vi "Tag Frames.vi"(5 "Single Channel Select":T5(ring), 6 "Frame Tag Bypass":T1, 7 "Enable Frame Tagging":bool, 8 "Input Valid":bool, 9 "Line Status In":T3, 10 "DC Overvoltage":bool, 11 "Data In":i16[](array[numeric])=[0, 0, 0, 0]) -> (1 "Line Status Out":T3, 3 "Data":T4, 4 "Frames Acquired":u32)   [LabVIEW 2014]
uses:
  Acquisition Engine/Acquisition Status.ctl
  Async Frametag Data.ctl
panel:
  # "Copyright 2014 Vidrio Technologies\nScanImage 5 software is licensed under the Apache License, Version 2.0 (the \"License\"); you may not use any files contained\nwithin the ScanImage 5 release except in compliance with the License. You may obtain a copy of the License at\n http://www.apache.org/licenses/LICENSE-2.0\nUnless required by applicable law or agreed to in writing, software distributed under the License is distributed on an\n\"AS IS\" BASIS, WITHOUT WARRANTIES OR CONDITIONS OF ANY KIND, either express or implied. See the License for the\n specific language governing permissions and limitations under the License."
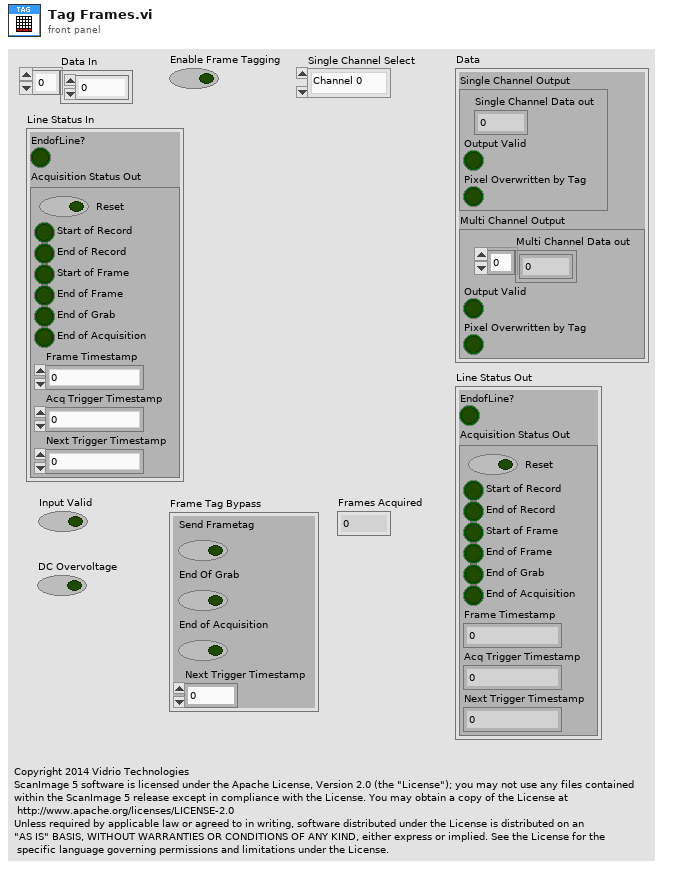
[diagram p1: front panel]
types:
  T1 = typedef "Async Frametag Data.ctl" = cluster{"Send Frametag":bool, "End Of Grab":bool, "End of Acquisition":bool, "Next Trigger Timestamp":u64}
  T2 = typedef "Acquisition Status.ctl" = cluster{"Reset":bool, "Start of Record":bool, "End of Record":bool, "Start of Frame":bool, "End of Frame":bool, "End of Grab":bool, "End of Acquisition":bool, "Frame Timestamp":u64, "Acq Trigger Timestamp":u64, "Next Trigger Timestamp":u64}
  T3 = cluster{"EndofLine?":bool, "Acquisition Status Out":T2}
  T4 = cluster{"Single Channel Output":cluster{"Single Channel Data out":i16, "Output Valid":bool, "Pixel Overwritten by Tag":bool}, "Multi Channel Output":cluster{"Multi Channel Data out":i16[], "Output Valid":bool, "Pixel Overwritten by Tag":bool}}
  T5 = enum8{"Channel 0", "Channel 1", "Channel 2", "Channel 3"}
  T6 = cluster{"Multi Channel Data out":i16[], "Output Valid":bool, "Pixel Overwritten by Tag":bool}
  T7 = cluster{"Single Channel Data out":i16, "Output Valid":bool, "Pixel Overwritten by Tag":bool}
  T8 = typedef "Frametag Data.ctl" = cluster{"Acquisition Status Flags":u16, "Frame Number":u32, "Frame Timestamp":u64, "Acq Trigger Timestamp":u64, "Next Trigger Timestamp":u64}
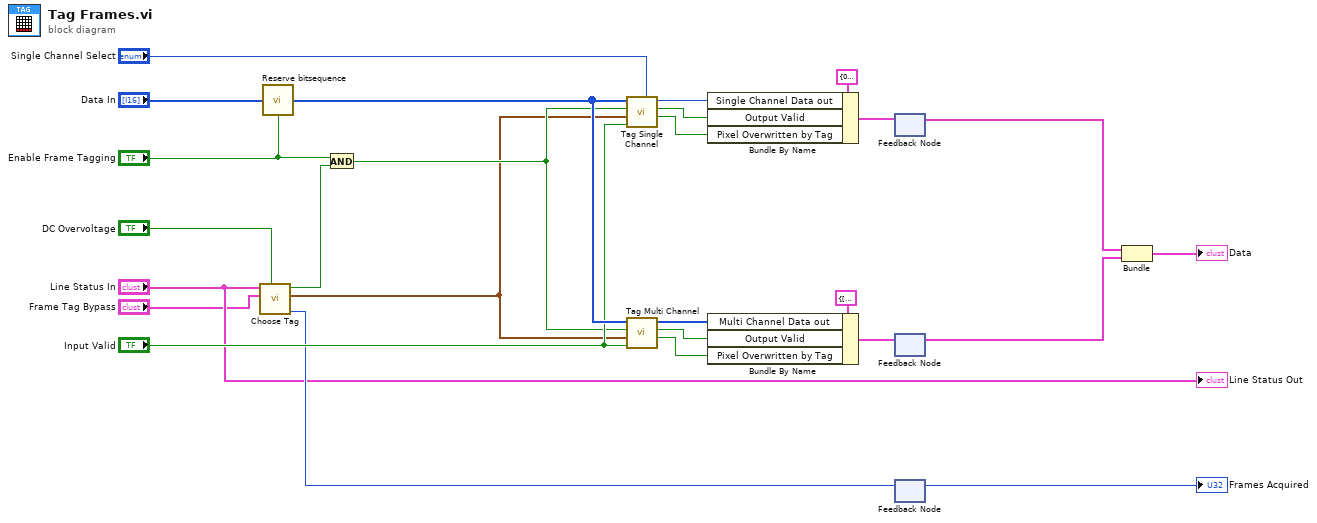
[diagram p0: block diagram]
diagram:
  n1 = call "Choose Tag.vi"("DC Overvoltage"="DC Overvoltage", "Frame Tag Bypass"="Frame Tag Bypass", "Line Status In"="Line Status In") -> ("Frame Count"=w8:u32, "Frametag Data"=w1:T8, "Send Tag"=w3:bool)  [unwired: 6 in]
  n2 = call "Reserve bitsequence.vi"("Data in"="Data In", "Reserve bitsequence"="Enable Frame Tagging") -> ("Data out"=w26:i16[])  [unwired: 13 in]
  n3 = And(x="Enable Frame Tagging", y=w3) -> (x .and. y?=w2:bool)
  n4 = call "Tag Single Channel.vi"("Data in"=w26, "Tag Record"=w2, "TagData"=w1, "Input Valid"="Input Valid", "Channel"="Single Channel Select") -> ("Single Channel Data out"=w22:i16, "Output Valid"=w21:bool, "Pixel Overwritten by Tag"=w23:bool)  [unwired: 3 in]
  n5 = call "Tag Multi Channel.vi"("Data in"=w26, "Tag Record"=w2, "TagData"=w1, "Input Valid"="Input Valid") -> ("Data out"=w18:i16[], "Output Valid"=w17:bool, "Pixel Overwritten"=w16:bool)  [unwired: 4 in]
  n6 = Bundle By Name(cluster=T7 {"Single Channel Data out"=0, "Output Valid"=FALSE, "Pixel Overwritten by Tag"=FALSE} ("Single Channel Output"), "Single Channel Data out"=w22, "Output Valid"=w21, "Pixel Overwritten by Tag"=w23) -> (w14:T7)
  n7 = Bundle By Name(cluster=T6 {"Multi Channel Data out"=[0, 0, 0, 0], "Output Valid"=FALSE, "Pixel Overwritten by Tag"=FALSE} ("Multi Channel Output"), "Multi Channel Data out"=w18, "Output Valid"=w17, "Pixel Overwritten by Tag"=w16) -> (w15:T6)
  n8 = feedback-in #1(w14) -> ()
  n9 = feedback #1() -> (w13:T7)  [unwired: 1 in]
  n10 = feedback #2() -> (w12:T6)  [unwired: 1 in]
  n11 = feedback-in #2(w15) -> ()
  n12 = feedback #3() -> (→"Frames Acquired":u32)  [unwired: 1 in]
  n13 = feedback-in #3(w8) -> ()
  n14 = Bundle("Single Channel Output"=w13, "Multi Channel Output"=w12) -> (→"Data":T4)  [unwired: 1 in]
  "Line Status Out" <- "Line Status In"
